vi "beginReceiveHealthAndStatus.vi"(8 "error in (no error)":errorcluster, 11 "Model in":refnum<class "Model.lvclass">) -> (0 "error out":errorcluster, 3 "Model out":refnum<class "Model.lvclass">)   [LabVIEW 2016, in "Model.lvclass"]
uses:
  Model.lvclass
  Model.lvclass/Model.ctl
  Common_RT_HealthAndStatus/RTHealthAndStatus/RTHealthAndStatus.lvclass
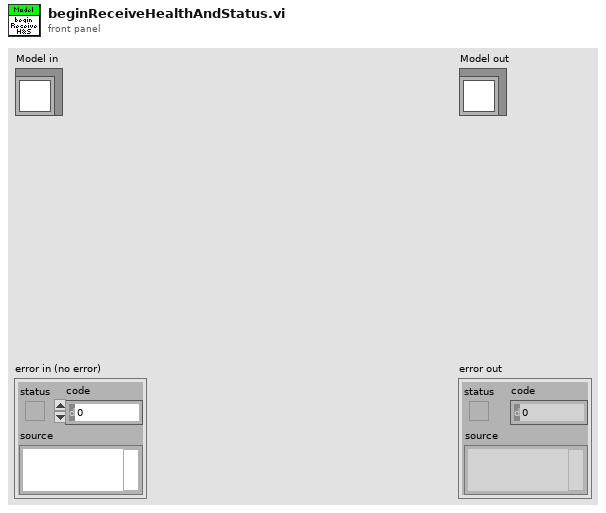
[diagram p1: front panel]
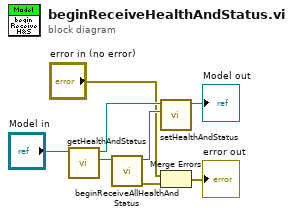
[diagram p0: block diagram]
diagram:
  n1 = call "getHealthAndStatus.vi"("Model in"="Model in") -> ("HealthAndStatus"=w8:refnum<class "RTHealthAndStatus.lvclass">, "Model out"=w6:refnum<class "Model.lvclass">)  [unwired: 9 in]
  n2 = call "beginReceiveAllHealthAndStatus.vi"("RTHealthAndStatus in"=w8) -> ("error out"=w3:errorcluster, "RTHealthAndStatus out"=w7:refnum<class "RTHealthAndStatus.lvclass">)  [unwired: 9 in]
  n3 = call "setHealthAndStatus.vi"("HealthAndStatus"=w7, "Model in"=w6) -> ("Model out"=→"Model out":refnum<class "Model.lvclass">)  [unwired: 9 in]
  n4 = Merge Errors("error in (no error)", w3) -> (→"error out":errorcluster)
